vi "qUSG CMD.vi"(0 "System no.":i32=1 min=1 max=4 step=1, 2 "Command":string, 5 "error in":errorcluster) -> (14 "Array of CommandInfo":T1[](array[typedef]), 19 "error out":errorcluster)   [LabVIEW 2026]
doc: "USG? CMD (Command Overview)\n\nDescription\nOutputs the \"CMD\" section of the user guide.\nDepending on the argument used, either all commands supported by the controller are listed or \nan individual command is described in more detail.\n\nFormat\nUSG? CMD[ <Command>]\n\nArguments\n<Command>\nCommand for which information is to be queried.\nPossible values:\n- Command mnemonics listed in the response to USG? CMD in the <Command> field.\n- Section commands (p. 86): \nFor commands whose first argument is <Section>, a keyword, i.e. a possible value for \n<Section>, can be entered after the command mnemonic. Command mnemonic and \nkeyword must be separated by a space. The possible keywords are listed in the <Name> \nfield in the response to USG? CMD <Command>. See example 2 in the description of the \nresponse.\n\nResponse\nUSG? CMD without additional arguments outputs a list of all commands that can be executed in \nthe current user command level (p. 69). Output format:\nThe Command Overview block consists of at least the following fields:\n- Command Command mnemonic\n- Arguments Syntax for the arguments of the command. The value \"-\" means that the \ncommand does not have any arguments.\n- Description Description of the command\nUSG? CMD <Command> outputs information on the command specified in <Command>. \nDepending on the command, the \"Command Overview\" block may contain subblocks.\nExample 1: View USG? CMD for the UCL command (p. 69) \n>>usg? cmd ucl\n<<#Command Overview: <Command> <Arguments> <Description>\n<<UCL <USR> [<PWD>] Set User Command Level\n<< #Related Units: <Container Unit> <Function Unit>\n<< SYS_1 INTPR_1\n<< #END Related Units\n<<#END Command Overview\nExample 2: View USG? CMD for the REC section command (p. 34) \nWhat are the keywords for the REC section command, and what do they mean? The keywords \nare queried with USG? CMD REC:\n>>usg? cmd rec\n<<#Command Overview: <Command> <Arguments> <Description>\n<<REC <Section> Data recorder related commands\n<< #Section: <Name> <Description>\n<< RATE Set recording rate [no. of servo cycles]\n<< START Start the recorder\n<< STOP Stop the recorder\n<< TRACE Specify parameter to be recorded\n<< TRG Configure trigger for start of recording\n<< #END Section\n<<#END Command Overview\nOne keyword for REC is, for example, \"TRG\" for the trigger configuration of the data recorder. \nDetails are queried with USG? CMD REC TRG: \n>>usg? cmd rec trg\n<<#Command Overview: <Command> <Arguments> <Description>\n<<REC TRG <RecorderID> <RecorderTrigger> [<TriggerOption1>\n[<TriggerOption2>]] Configure trigger for start of recording\n<< #Related Units: <Container Unit> <Function Unit>\n<< REC_1 -\n<< REC_2 -\n<< #END Related Units\n<<#END Command Overview\nPlease note: Trigger options, states of the data recorder, etc. are properties of the data \nrecorders and thus queried with USG? PROP (p. 79). \n\nNotes\nUSG? without any arguments (p. 72) displays the contents of the user guide, i.e. the titles of the \navailable sections.\nUSG? CMD is comparable to HLP? (p. 18) from GCS 2.0, but it is not identical to this command.\n\nUser command level\nUSR"
uses:
  CommandInfo.ctl
  <vilib>/Utility/error.llb/Trim Whitespace One-Sided.vi
panel:
  # "USG? CMD (Command Overview)\n\nOutputs the \"CMD\" section of the user guide.\nDepending on the argument used, either all commands supported by the controller are listed or \nan individual command is described in more detail."
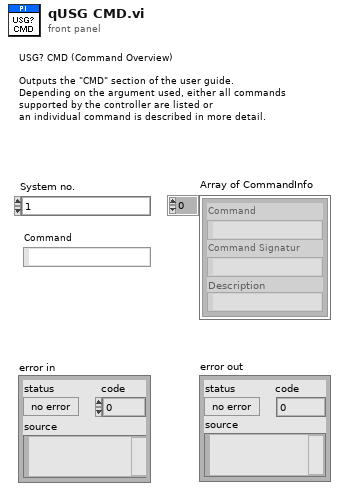
[diagram p1: front panel]
types:
  T1 = typedef "CommandInfo.ctl" = cluster{"Command":string, "Command Signatur":string, "Description":string}
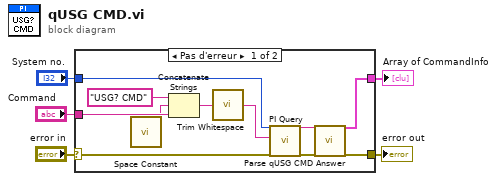
[diagram p0: block diagram]
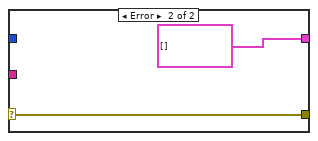
[diagram p2: hidden frame]
diagram:
  n1 = case shown="Pas d'erreur" "error in" {
    selector: "error in" -> [w16 w18]
    tunnel: "System no." -> [w15 _]
    tunnel: [w11 w18] -> w4
    tunnel: [w10 T1[] [] ("Array of ParametersInfo")] -> w2
    tunnel: "Command" -> [w8 _]
    frame No Error {
      n2 = call <vilib>:"Space Constant.vi"() -> ("String"=w7:string)
      n3 = Concatenate Strings("USG? CMD", w7, w8) -> (w9:string)
      n4 = call <vilib>:"Trim Whitespace.vi"("string"=w9) -> ("trimmed string"=w6:string)  [unwired: 1 in]
      n5 = call "PI Query.vi"("System no."=w15, "String to send"=w6, "error in"=w16) -> ("String read"=w13:string, "error out"=w12:errorcluster)  [unwired: 13 in, 2 out]
      n6 = call "Parse qUSG CMD Answer.vi"("Answer To Parse"=w13, "error in"=w12) -> ("Array of CommandInfo"=w10:T1[], "error out"=w11:errorcluster)  [unwired: 16 in]
    }
    frame Error {
    }
  }
  "error out" <- w4
  "Array of CommandInfo" <- w2
